vi "ProduceAcceptKey.vi"(11 "Sec-WebSocket-Key":string) -> (3 "Sec-WebSocket-Accept":string)   [LabVIEW 2016, in "WebSockets.lvlib"]
doc: "Generates the WebSockets Accept key for the HTTP handshaking response. This is a base-64 encoding + SHA-1 of the received key and the WebSockets magic string.\nWebSockets 1.6.0.22\nSam Sharp - MediaMongrels Ltd\nCopyright (c) 2016, MediaMongrels Ltd"
uses:
  WebSockets.lvlib
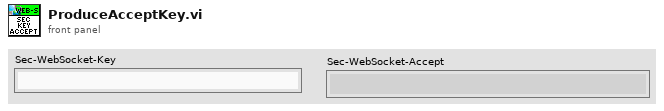
[diagram p1: front panel]
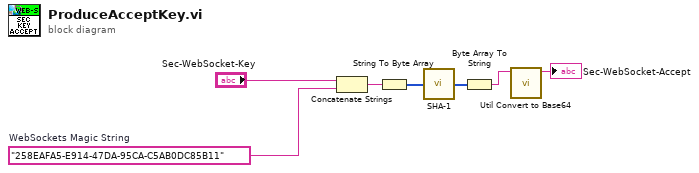
[diagram p0: block diagram]
diagram:
  w6 = "258EAFA5-E914-47DA-95CA-C5AB0DC85B11"  # WebSockets Magic String
  n1 = Concatenate Strings("Sec-WebSocket-Key", w6) -> (w5:string)
  n2 = String To Byte Array(string=w5) -> (unsigned byte array=w4:u8[])
  n3 = call "SHA-1.vi"("Data"=w4) -> ("message-digest"=w3:u8[])
  n4 = Byte Array To String(unsigned byte array=w3) -> (string=w2:string)
  n5 = call "Util Convert to Base64.vi"("String"=w2) -> ("Base64 String"=→"Sec-WebSocket-Accept":string)  [unwired: 10 in]
